vi "Load User Devices.vi"(8 "error in (no error)":errorcluster, 11 "App in":refnum<class "App.lvclass">) -> (0 "error out":errorcluster, 3 "App out":refnum<class "App.lvclass">)   [LabVIEW 2020, in "PicoG-App.lvlib" / "App.lvclass"]
uses:
  App.lvclass
  DeviceListPanel/DeviceListPanel.lvclass
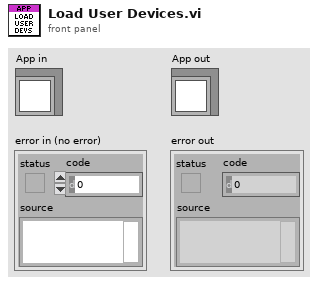
[diagram p1: front panel]
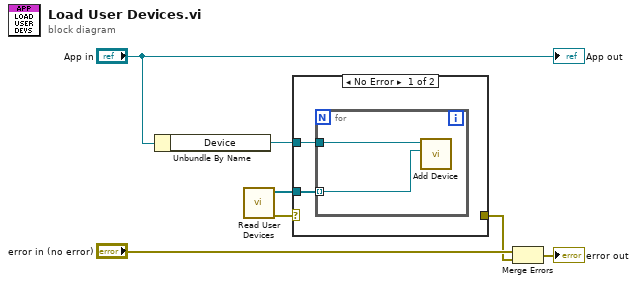
[diagram p0: block diagram]
diagram:
  n1 = Unbundle By Name("App in") -> ("Device"=w3:refnum<class "DeviceListPanel.lvclass">)
  n2 = call "Read User Devices.vi"() -> ("error out"=w5:errorcluster, "User Devices"=w4:refnum<class "Device.lvclass">[])  [unwired: 10 in]
  n3 = case shown="No Error" w5 {
    selector: w5 -> [_ w12]
    tunnel: w4 -> [w8 _]
    tunnel: w3 -> [w9 _]
    tunnel: [_ w12] -> w1
    frame No Error {
      n4 = for {
        tunnel: w9 -> [w11]
        tunnel: w8 -> [w10] mode=indexing
        n5 = call "Add Device.vi"("Device"=w10, "DeviceListPanel in"=w11) -> ()  [unwired: 8 in, 2 out]
      }
    }
    frame Error {
    }
  }
  n6 = Merge Errors("error in (no error)", w1) -> (→"error out":errorcluster)
  "App out" <- "App in"
